vi "StopAcquisitionRequest.vi"(8 "error in (no error)":errorcluster, 11 "ModuleID":i32) -> (0 "error out":errorcluster)   [LabVIEW 2018, in "ScopeModule.lvlib"]
uses:
  ScopeModule.lvlib
  ScopeShared/clEventType.ctl
  <vilib>/Utility/error.llb/Error Cluster From Error Code.vi
  <vilib>/ErrorRing/Error Ring.xnode
  ScopeShared/ScopeShared.lvlib
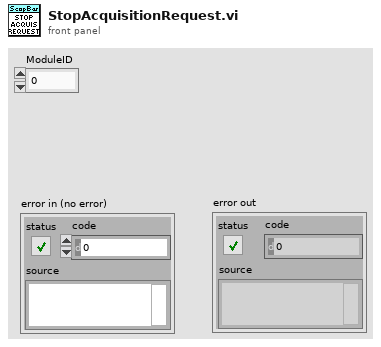
[diagram p1: front panel]
types:
  T1 = typedef "ScopeShared.lvlib/clRequestEvents.ctl" = cluster{"StopRequest":refnum<user-event>, "PathToINI":refnum<user-event>, " LoadPlugin":refnum<user-event>, "ShowPanel":refnum<user-event>, "Abort":refnum<user-event>, "SetAcquisition":refnum<user-event>, "SetChannel":refnum<user-event>, "SetTrigger":refnum<user-event>, "GetAcquisition":refnum<user-event>, "GetChannel":refnum<user-event>, "GetTrigger":refnum<user-event>, "FetchWaveform":refnum<user-event>, "InitAcquisition":refnum<user-event>, "ReadWaveform":refnum<user-event>, "GetHandle":refnum<user-event>, "SetHandle":refnum<user-event>, "GetModel":refnum<user-event>, "SetModel":refnum<user-event>, "ConfigAquisition":refnum<user-event>, "ConfigChannels":refnum<user-event>, "ConfigTrigger":refnum<user-event>, "Initialize":refnum<user-event>, "SetExtAcquisition":refnum<user-event>, "StopAcquisition":refnum<user-event>, "PrefDlg":refnum<user-event>, "Close":refnum<user-event>, "SetSync":refnum<user-event>}
  T2 = typedef "ScopeShared.lvlib/clEventType.ctl" = cluster{"ModuleID":i32, "Data":variant}
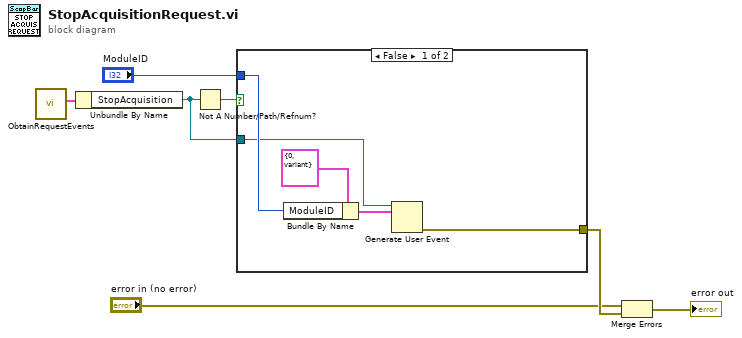
[diagram p0: block diagram]
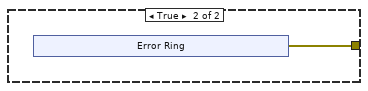
[diagram p2: hidden frame]
diagram:
  n1 = call "ObtainRequestEvents.vi"() -> ("ScopeRequests"=w7:T1)  [unwired: 10 in, 1 out]
  n2 = Unbundle By Name(w7) -> ("StopAcquisition"=w5:refnum<user-event>)
  n3 = Not A Number/Path/Refnum?(number/path/refnum=w5) -> (NaN/Path/Refnum?=w6:bool)
  n4 = case shown="False" w6 {
    tunnel: w5 -> [w9 _]
    tunnel: "ModuleID" -> [w11 _]
    tunnel: [w8 w13] -> w2
    frame False {
      n5 = Bundle By Name(cluster=T2 {"ModuleID"=0, "Data"=variant} ("clEventType"), "ModuleID"=w11) -> (w10:T2)
      n6 = Generate User Event(user event=w9, event data cluster=w10) -> (error out=w8:errorcluster)  [unwired: 2 in, 1 out]
    }
    frame True {
      n7 = xnode "Error Ring"() -> ("error out"=w13:errorcluster)
    }
  }
  n8 = Merge Errors("error in (no error)", w2) -> (→"error out":errorcluster)
